vi "Search_ERD_JSON.vi"(0 "ERD Number":u16, 7 "JSON Text":string, 11 "error in":errorcluster) -> (4 "ERD":string, 15 "error out":errorcluster)   [LabVIEW 2021]
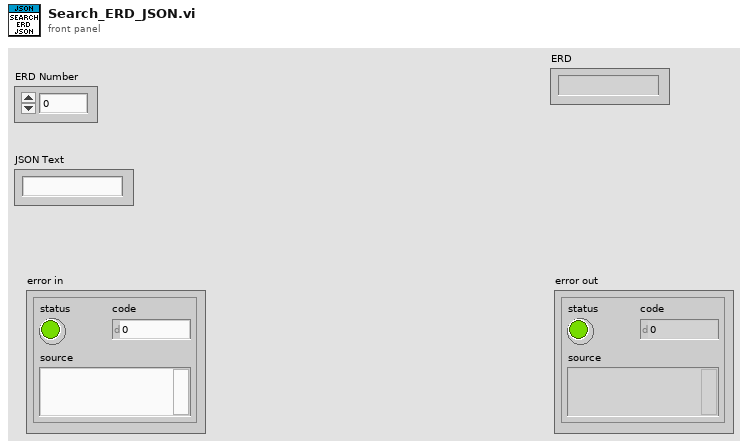
[diagram p1: front panel]
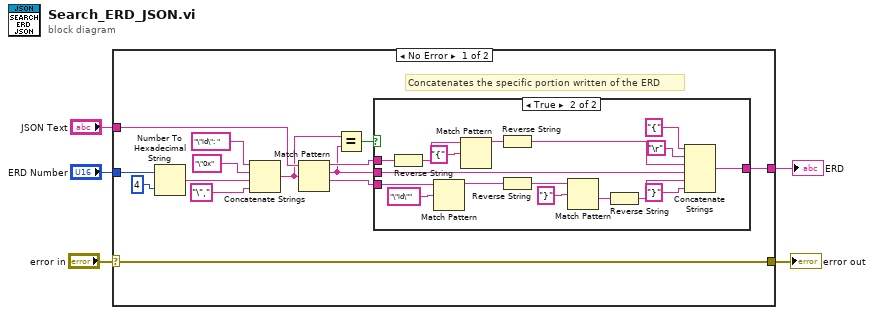
[diagram p0: block diagram]
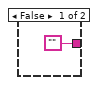
[diagram p2: hidden frame]
diagram:
  n1 = case shown="No Error" "error in" {
    selector: "error in" -> [w8 w38]
    tunnel: "JSON Text" -> [w11 _]
    tunnel: "ERD Number" -> [w10 _]
    tunnel: [w9 _] -> w3
    tunnel: [w8 w38] -> w1
    frame No Error {
      # "Concatenates the specific portion written of the ERD"
      n2 = Number To Hexadecimal String(1:i16 4 ("width (-)"), 2:w10) -> (0:w17:string)
      n3 = Concatenate Strings("\"id\": " ("string"), "\"0x" ("string"), w17, "\"," ("string")) -> (w7:string)
      n4 = Match Pattern(string=w11, regular expression=w7) -> (before substring=w14:string, match substring=w6:string, after substring=w13:string)  [unwired: 1 in, 1 out]
      n5 = Equal?(x=w7, y=w6) -> (x = y?=w12:bool)
      n6 = case shown="True" w12 {
        tunnel: ["" w24] -> w9
        tunnel: w14 -> [_ w23]
        tunnel: w6 -> [_ w22]
        tunnel: w13 -> [_ w21]
        frame False {
        }
        frame True {
          n7 = Reverse String(1:w23) -> (0:w31:string)
          n8 = Match Pattern(string=w21, regular expression="\"id\"") -> (before substring=w35:string)  [unwired: 1 in, 3 out]
          n9 = Match Pattern(string=w31, regular expression="{") -> (before substring=w29:string)  [unwired: 1 in, 3 out]
          n10 = Reverse String(1:w29) -> (0:w28:string)
          n11 = Reverse String(1:w35) -> (0:w34:string)
          n12 = Match Pattern(string=w34, regular expression="}") -> (after substring=w33:string)  [unwired: 1 in, 3 out]
          n13 = Reverse String(1:w33) -> (0:w32:string)
          n14 = Concatenate Strings("{" ("string"), "\r", w28, w22, w32, "}" ("string")) -> (w24:string)
        }
      }
    }
    frame Error {
    }
  }
  "ERD" <- w3
  "error out" <- w1
